vi "Retrieve Sample from Container.vi"(8 "error in (no error)":errorcluster, 9 "timeout in ms (1000)":i32=1000, 10 "Container":T1(ring)=enum."He Line", 11 "Transfer Line in":refnum<class "Transfer Line.lvclass">) -> (0 "error out":errorcluster, 2 "Sample out":refnum<class "Sample.lvclass">, 3 "Transfer Line out":refnum<class "Transfer Line.lvclass">)   [LabVIEW 2015, in "cRIO-Carbondioxide.lvlib" / "CO2-Actor.lvlib" / "Transfer Line.lvclass"]
uses:
  Actors/Transfer Line/Transfer Line.lvclass
  Sample/Sample.lvclass
  Actors/Transfer Line/Transfer Line.lvclass/Transfer Line.ctl
  Actors/Sample Line/Sample Line.lvclass
  Actors/CO2 Actor Messages/Ping Msg/Ping Msg.lvclass/Ping Msg.ctl
  <vilib>/ActorFramework/Message Enqueuer/Message Enqueuer.lvclass/Message Enqueuer.ctl
  Actors/Storage Line/Storage Line.lvclass
  Actors/Storage Line/Storage Line.lvclass/Storage Line.ctl
  Actors/Syringe Line/Syringe Line.lvclass
  Actors/Preparation Line/Preparation Line.lvclass
  Actors/He Line/He Line.lvclass
  Actors/He Line/He Line.lvclass/He Line.ctl
  <vilib>/ActorFramework/Message Enqueuer/Enqueue.vi
  Sample/Read Sample From Container.vi
  <vilib>/ActorFramework/Message Priority Queue/Priority Enqueue.vi
  Actors/CO2 Actor Messages/Ping Msg/Ping Msg.lvclass
  <vilib>/ActorFramework/Actor/Actor.lvclass
  Actors/CO2 Actor/CO2 Actor.lvclass
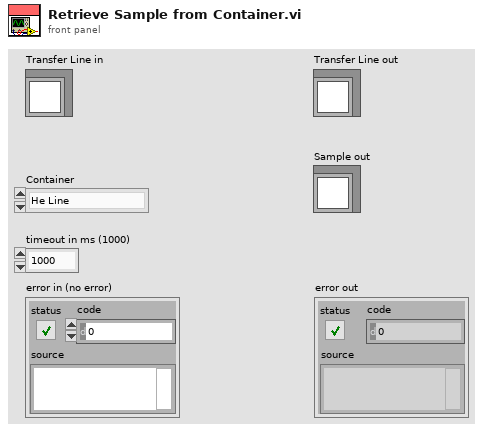
[diagram p1: front panel]
types:
  T1 = enum16{"None", "Sample Line", "Storage Line", "Syringe", "Preparation Line", "Transfer Line", "He Line"}
  T2 = typedef "Dedicated Enqueuers.ctl" = cluster{"Freezers":cluster{"Syringe":refnum<class "Message Enqueuer.lvclass">, "Tank 1":refnum<class "Message Enqueuer.lvclass">, "Tank 2":refnum<class "Message Enqueuer.lvclass">, "Tank 3":refnum<class "Message Enqueuer.lvclass">, "Tank 4":refnum<class "Message Enqueuer.lvclass">}, "Heaters":cluster{"Syringe":refnum<class "Message Enqueuer.lvclass">, "Piston":refnum<class "Message Enqueuer.lvclass">}, "Blowers":cluster{"Tank 1":refnum<class "Message Enqueuer.lvclass">, "Tank 2":refnum<class "Message Enqueuer.lvclass">, "Tank 3":refnum<class "Message Enqueuer.lvclass">, "Tank 4":refnum<class "Message Enqueuer.lvclass">, "Syringe":refnum<class "Message Enqueuer.lvclass">}, "Sample Line":refnum<class "Message Enqueuer.lvclass">, "Storage Line":refnum<class "Message Enqueuer.lvclass">, "Transfer Line":refnum<class "Message Enqueuer.lvclass">, "Syringe Stepper":refnum<class "Message Enqueuer.lvclass">, "Syringe Line":refnum<class "Message Enqueuer.lvclass">, "Capillary Line":refnum<class "Message Enqueuer.lvclass">, "Preparation Line":refnum<class "Message Enqueuer.lvclass">, "Turbo":refnum<class "Message Enqueuer.lvclass">, "Vacuum":refnum<class "Message Enqueuer.lvclass">, "He Line":refnum<class "Message Enqueuer.lvclass">, "Cylinder":refnum<class "Message Enqueuer.lvclass">}
  T3 = typedef "Sample Line State Enumerator.ctl" = enum16{"All lines closed", "Sample line 1.", "Sample line 2.", "Sample line 3.", "Sample line 4.", "Sample line 5.", "Out of range"}
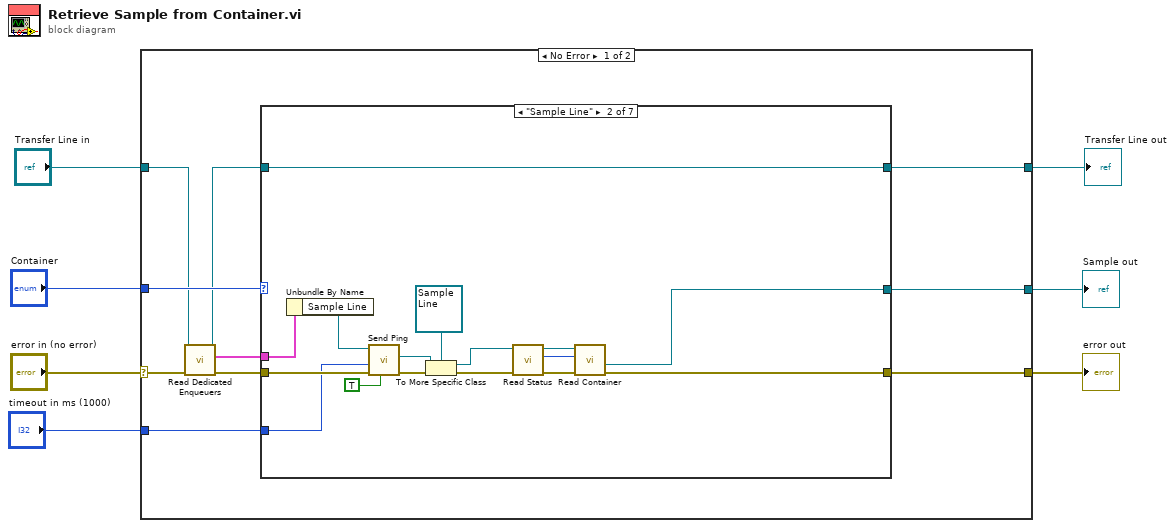
[diagram p0: block diagram]
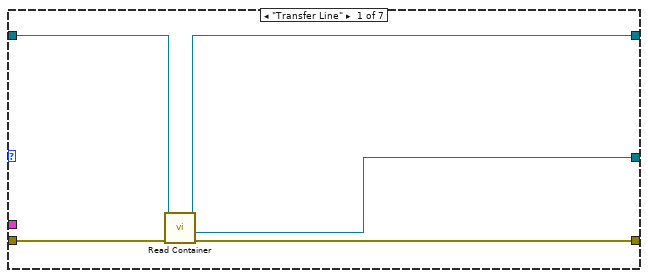
[diagram p2: hidden frame]
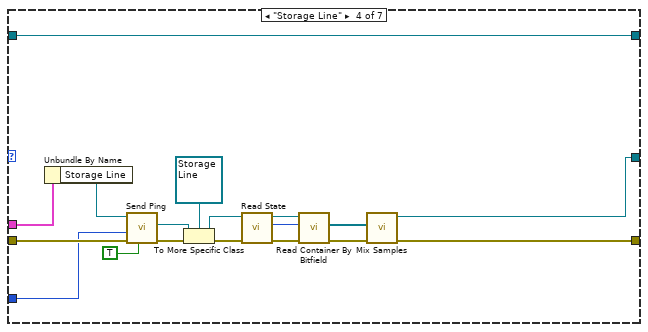
[diagram p4: hidden frame]
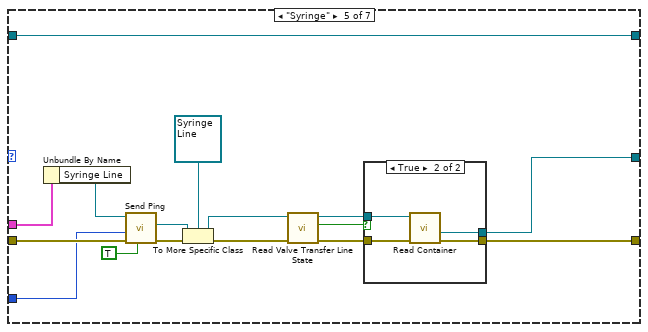
[diagram p5: hidden frame]
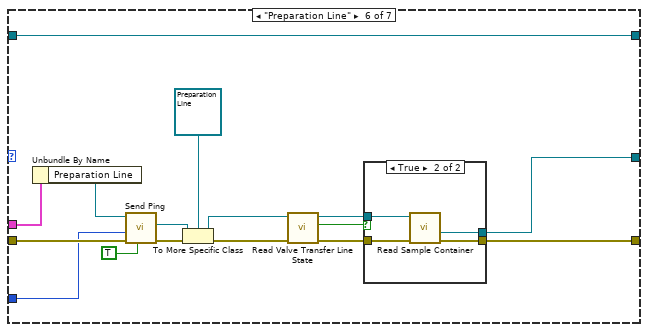
[diagram p7: hidden frame]
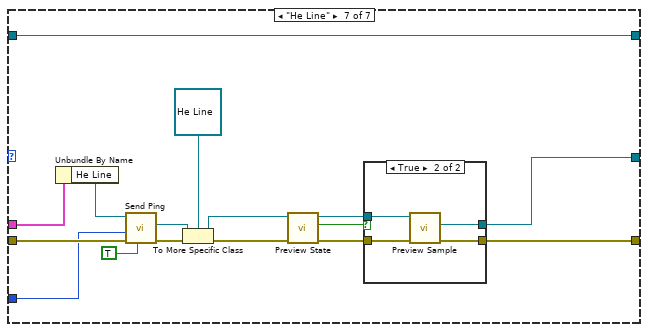
[diagram p9: hidden frame]
diagram:
  n1 = case shown="No Error" "error in (no error)" {
    selector: "error in (no error)" -> [w13 w123]
    tunnel: [w15 w123] -> w6
    tunnel: "Container" -> [w17 _]
    tunnel: [w14 _] -> w4
    tunnel: "Transfer Line in" -> [w11 w122]
    tunnel: [w16 w122] -> w2
    tunnel: "timeout in ms (1000)" -> [w8 _]
    frame No Error {
      n2 = call "Read Dedicated Enqueuers.vi"("error in (no error)"=w13, "CO2 Actor in"=w11) -> ("error out"=w12:errorcluster, "Dedicated Enqueuers"=w9:T2, "CO2 Actor out"=w10:refnum<class "Transfer Line.lvclass">)  [unwired: 6 in, 1 out]
      n3 = case shown="\"Sample Line\"" w17 {
        tunnel: w12 -> [w22 w37 w40 w54 w71 w92 w113]
        tunnel: [w19 w26 w40 w43 w66 w88 w109] -> w15
        tunnel: w10 -> [w21 w24 w39 w42 w65 w87 w108]
        tunnel: [w20 w24 w39 w42 w65 w87 w108] -> w16
        tunnel: [w18 w25 _ w44 w67 w89 w110] -> w14
        tunnel: w9 -> [_ w38 _ w53 w70 w91 w112]
        tunnel: w8 -> [_ w23 _ w41 w59 w80 w101]
        frame "Transfer Line" {
          n4 = call "Read Container.vi"("error in (no error)"=w22, "Transfer Line in"=w21) -> ("error out"=w19:errorcluster, "Sample"=w18:refnum<class "Sample.lvclass">, "Transfer Line out"=w20:refnum<class "Transfer Line.lvclass">)  [unwired: 5 in, 2 out]
        }
        frame "Sample Line" {
          n5 = Unbundle By Name(w38) -> ("Sample Line"=w36:refnum<class "Message Enqueuer.lvclass">)
          n6 = call "Send Ping.vi"("Return Self (F)"=TRUE, "error in (no error)"=w37, "timeout in ms (1000)"=w23, "Message Enqueuer"=w36) -> ("error out"=w34:errorcluster, "Actor out"=w31:refnum<class "Actor.lvclass">)  [unwired: 4 in, 2 out]
          n7 = To More Specific Class(target class=refnum<class "Sample Line.lvclass"> refnum ("Sample Line in"), reference=w31, error in=w34) -> (specific class reference=w30:refnum<class "Sample Line.lvclass">, error out=w33:errorcluster)
          n8 = call "Read Status.vi"("error in (no error)"=w33, "Sample Line in"=w30) -> ("error out"=w29:errorcluster, "Status"=w27:T3, "Sample Line out"=w28:refnum<class "Sample Line.lvclass">)  [unwired: 7 in]
          n9 = call "Read Container.vi"("error in (no error)"=w29, "Sample Line (All Closed)"=w27, "Sample Line in"=w28) -> ("error out"=w26:errorcluster, "Sample"=w25:refnum<class "Sample.lvclass">)  [unwired: 5 in, 2 out]
        }
        frame "None", Default {
        }
        frame "Storage Line" {
          n10 = Unbundle By Name(w53) -> ("Storage Line"=w58:refnum<class "Message Enqueuer.lvclass">)
          n11 = call "Send Ping.vi"("Return Self (F)"=TRUE, "error in (no error)"=w54, "timeout in ms (1000)"=w41, "Message Enqueuer"=w58) -> ("error out"=w56:errorcluster, "Actor out"=w55:refnum<class "Actor.lvclass">)  [unwired: 4 in, 2 out]
          n12 = To More Specific Class(target class=refnum<class "Storage Line.lvclass"> refnum ("Storage Line in"), reference=w55, error in=w56) -> (specific class reference=w50:refnum<class "Storage Line.lvclass">, error out=w52:errorcluster)
          n13 = call "Read State.vi"("error in (no error)"=w52, "Storage Line in"=w50) -> ("error out"=w49:errorcluster, "State"=w48:u16, "Storage Line out"=w47:refnum<class "Storage Line.lvclass">)  [unwired: 5 in, 2 out]
          n14 = call "Read Container By Bitfield.vi"("error in (no error)"=w49, "Bitfield"=w48, "Storage Line in"=w47) -> ("error out"=w46:errorcluster, "Samples"=w45:refnum<class "Sample.lvclass">[])  [unwired: 4 in, 3 out]
          n15 = call "Mix Samples.vi"("error in (no error)"=w46, "Samples In"=w45) -> ("error out"=w43:errorcluster, "Sample out"=w44:refnum<class "Sample.lvclass">)  [unwired: 6 in, 2 out]
        }
        frame "Syringe" {
          n16 = Unbundle By Name(w70) -> ("Syringe Line"=w74:refnum<class "Message Enqueuer.lvclass">)
          n17 = call "Send Ping.vi"("Return Self (F)"=TRUE, "error in (no error)"=w71, "timeout in ms (1000)"=w59, "Message Enqueuer"=w74) -> ("error out"=w73:errorcluster, "Actor out"=w72:refnum<class "Actor.lvclass">)  [unwired: 4 in, 2 out]
          n18 = To More Specific Class(target class=refnum<class "Syringe Line.lvclass"> refnum ("Syringe Line in"), reference=w72, error in=w73) -> (specific class reference=w63:refnum<class "Syringe Line.lvclass">, error out=w64:errorcluster)
          n19 = call "Read Valve Transfer Line State.vi"("error in (no error)"=w64, "Syringe Line in"=w63) -> ("error out"=w62:errorcluster, "Open?"=w61:bool, "Syringe Line out"=w60:refnum<class "Syringe Line.lvclass">)  [unwired: 6 in, 1 out]
          n20 = case shown="True" w61 {
            tunnel: w62 -> [w75 w79]
            tunnel: [_ w78] -> w67
            tunnel: [w75 w77] -> w66
            tunnel: w60 -> [_ w76]
            frame False {
            }
            frame True {
              n21 = call "Read Container.vi"("error in (no error)"=w79, "Syringe Line in"=w76) -> ("error out"=w77:errorcluster, "Sample"=w78:refnum<class "Sample.lvclass">)  [unwired: 6 in, 2 out]
            }
          }
        }
        frame "Preparation Line" {
          n22 = Unbundle By Name(w91) -> ("Preparation Line"=w95:refnum<class "Message Enqueuer.lvclass">)
          n23 = call "Send Ping.vi"("Return Self (F)"=TRUE, "error in (no error)"=w92, "timeout in ms (1000)"=w80, "Message Enqueuer"=w95) -> ("error out"=w94:errorcluster, "Actor out"=w93:refnum<class "Actor.lvclass">)  [unwired: 4 in, 2 out]
          n24 = To More Specific Class(target class=refnum<class "Preparation Line.lvclass"> refnum ("Preparation Line in"), reference=w93, error in=w94) -> (specific class reference=w81:refnum<class "Preparation Line.lvclass">, error out=w86:errorcluster)
          n25 = call "Read Valve Transfer Line State.vi"("error in (no error)"=w86, "Preparation Line in"=w81) -> ("error out"=w85:errorcluster, "Open?"=w84:bool, "Preparation Line out"=w83:refnum<class "Preparation Line.lvclass">)  [unwired: 6 in, 1 out]
          n26 = case shown="True" w84 {
            tunnel: w85 -> [w96 w100]
            tunnel: [_ w99] -> w89
            tunnel: [w96 w98] -> w88
            tunnel: w83 -> [_ w97]
            frame False {
            }
            frame True {
              n27 = call "Read Sample Container.vi"("error in (no error)"=w100, "Preparation Line in"=w97) -> ("error out"=w98:errorcluster, "Sample"=w99:refnum<class "Sample.lvclass">)  [unwired: 6 in, 2 out]
            }
          }
        }
        frame "He Line" {
          n28 = Unbundle By Name(w112) -> ("He Line"=w116:refnum<class "Message Enqueuer.lvclass">)
          n29 = call "Send Ping.vi"("Return Self (F)"=TRUE, "error in (no error)"=w113, "timeout in ms (1000)"=w101, "Message Enqueuer"=w116) -> ("error out"=w115:errorcluster, "Actor out"=w114:refnum<class "Actor.lvclass">)  [unwired: 4 in, 2 out]
          n30 = To More Specific Class(target class=refnum<class "He Line.lvclass"> refnum ("Preparation Line in"), reference=w114, error in=w115) -> (specific class reference=w102:refnum<class "He Line.lvclass">, error out=w107:errorcluster)
          n31 = call "Preview State.vi"("error in (no error)"=w107, "He Line in"=w102) -> ("error out"=w106:errorcluster, "Is Open?"=w105:bool, "He Line out"=w104:refnum<class "He Line.lvclass">)  [unwired: 7 in]
          n32 = case shown="True" w105 {
            tunnel: w106 -> [w117 w121]
            tunnel: [_ w118] -> w110
            tunnel: [w117 w120] -> w109
            tunnel: w104 -> [_ w119]
            frame False {
            }
            frame True {
              n33 = call "Preview Sample.vi"("error in (no error)"=w121, "He Line in"=w119) -> ("error out"=w120:errorcluster, "element"=w118:refnum<class "Sample.lvclass">)  [unwired: 6 in, 2 out]
            }
          }
        }
      }
    }
    frame Error {
    }
  }
  "error out" <- w6
  "Sample out" <- w4
  "Transfer Line out" <- w2
